vi "DHE_SetDACsFile.vi"(2 "DHE_DACsFile":path) -> ()   [LabVIEW 2016]
uses:
  private/vis/DHE_VarAction.ctl
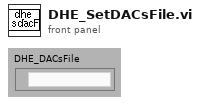
[diagram p1: front panel]
types:
  T1 = typedef "DHE_VarAction.ctl" = enum16{"read", "write"}
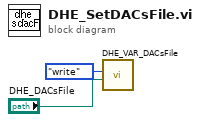
[diagram p0: block diagram]
diagram:
  n1 = call "DHE_VAR_DACsFile.vi"("value"="DHE_DACsFile", "action"=DHE_VarAction."write") -> ()  [unwired: 10 out]
